vi "Initialize.vi"(8 "error in (no error)":errorcluster, 11 "FLOM Settings in":T1={"VISA resource name"="", "Simulated?"=FALSE, "Pump Number"=1.0} {"Pump Number" min=1.0 max=20.0 step=1.0}) -> (0 "error out":errorcluster, 1 "Initialized":bool, 2 "No Pump Connected":bool, 3 "FLOM Settings out":T1={"VISA resource name"="", "Simulated?"=FALSE, "Pump Number"=1.0} {"Pump Number" min=1.0 max=20.0 step=1.0})   [LabVIEW 2018, in "FLOM Pump.lvlib"]
uses:
  FLOM Pump.lvlib
  Settings Cluster.ctl
  <vilib>/Instr/_visa.llb/VISA Configure Serial Port (Instr).vi
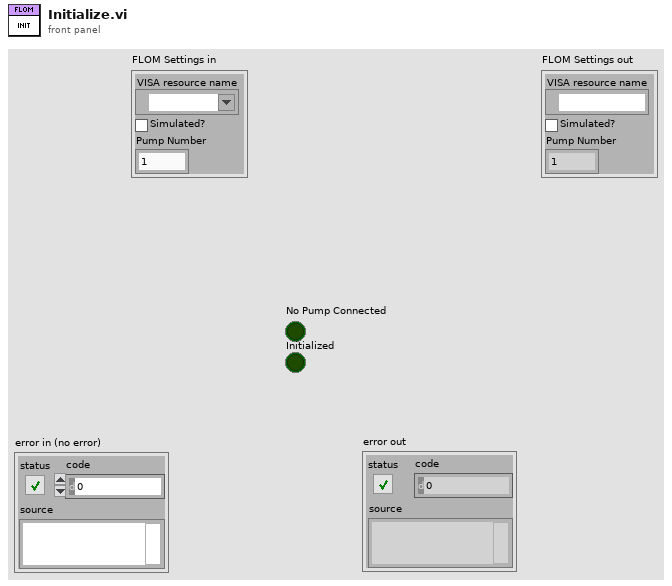
[diagram p1: front panel]
types:
  T1 = typedef "FLOM Pump.lvlib/Settings Cluster.ctl" = cluster{"VISA resource name":refnum<visa-resource-name>, "Simulated?":bool, "Pump Number":dbl}
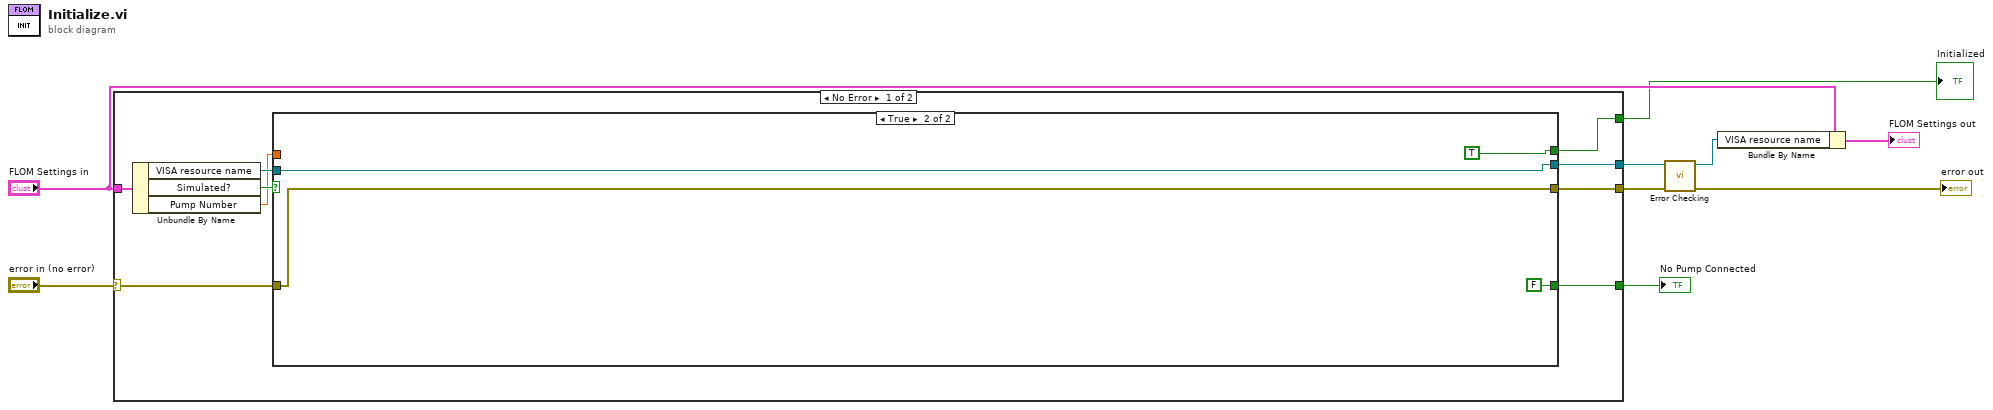
[diagram p0: block diagram]
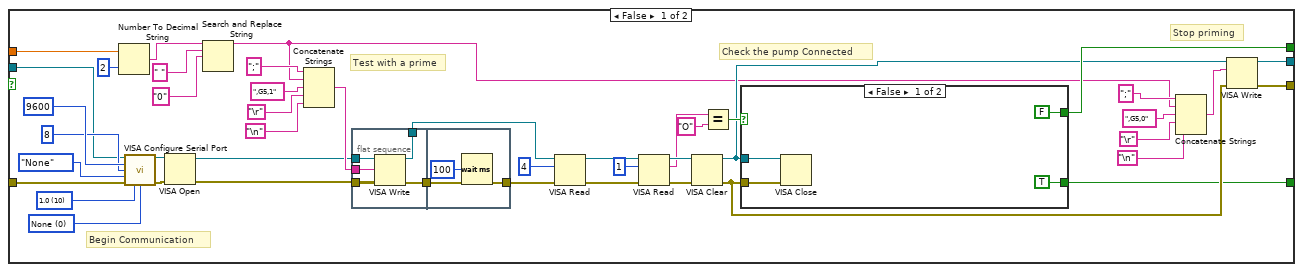
[diagram p2: hidden frame]
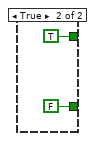
[diagram p3: hidden frame]
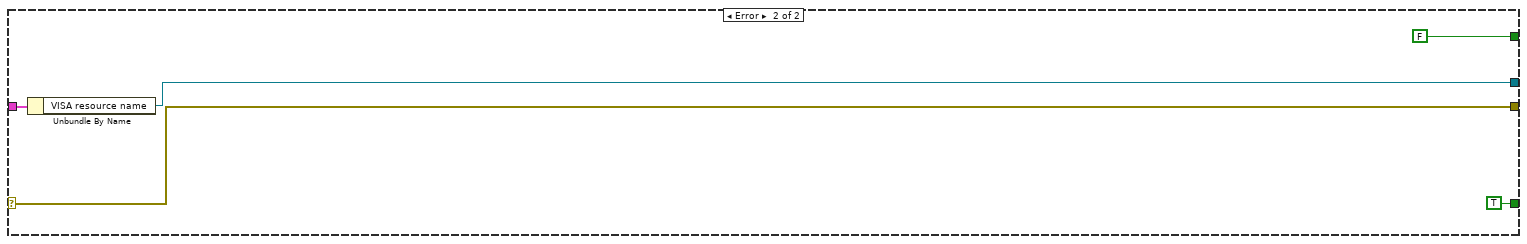
[diagram p4: hidden frame]
diagram:
  n1 = case shown="No Error" "error in (no error)" {
    selector: "error in (no error)" -> [w18 w85]
    tunnel: "FLOM Settings in" -> [w13 w84]
    tunnel: [w14 w85] -> w7
    tunnel: [w12 w83] -> w2
    tunnel: [w11 FALSE] -> w4
    tunnel: [w10 TRUE] -> w1
    frame No Error {
      n2 = Unbundle By Name(w13) -> ("VISA resource name"=w16:refnum<visa-resource-name>, "Simulated?"=w17:bool, "Pump Number"=w15:dbl)
      n3 = case shown="True" w17 {
        tunnel: w18 -> [w57 w80]
        tunnel: w16 -> [w55 w79]
        tunnel: w15 -> [w52 _]
        tunnel: [w22 w80] -> w14
        tunnel: [w20 w79] -> w12
        tunnel: [w47 TRUE] -> w11
        tunnel: [w19 FALSE] -> w10
        frame False {
          w59 = u16 0 items=["None", "XON/XOFF", "RTS/CTS", "XON/XOFF & RTS/CTS", "DTR/DSR", "XON/XOFF & DTR/DSR"] ("flow control (0:none)")
          w60 = u16 10 items=["1.0"=10, "1.5"=15, "2.0"=20] ("stop bits (10: 1 bit)")
          # "Stop priming"
          # "Test with a prime"
          # "Check the pump Connected"
          # "Begin Communication"
          n4 = Number To Decimal String(number=w52, width (-)=i16 2) -> (decimal integer string=w35:string)
          n5 = call-poly "VISA Configure Serial Port"("VISA resource name"=w55, "baud rate (9600)"=u32 9600, "data bits (8)"=u16 8, "parity (0:none)"=enum16{"None", "Odd", "Even", "Mark", "Space"}."None", "error in (no error)"=w57, "stop bits (10: 1 bit)"=w60, "flow control (0:none)"=w59) -> ("VISA resource name out"=w56:refnum<visa-resource-name>, "error out"=w58:errorcluster)  [unwired: 7 in]
          n6 = VISA Open(error in (no error)=w58, VISA resource name=w56) -> (VISA resource name=w31:refnum<visa-resource-name>, error out=w46:errorcluster)  [unwired: 3 in]
          n7 = Search and Replace String(input string=w35, search string=" ", replace string="0" ("replace string (\"\")")) -> (result string=w21:string)  [unwired: 5 in, 3 out]
          n8 = Concatenate Strings(";" ("string"), w21, ",G5,1" ("string"), "\r", "\n") -> (w53:string)
          n9 = flat-sequence {
            tunnel: w53 -> [w68]
            tunnel: w46 -> [w66]
            tunnel: [w67] -> w32
            tunnel: w31 -> [w65]
            tunnel: [w64] -> w30
            tunnel: [w70] -> w50
            tunnel: w32 -> [w70]
            frame #0 {
              n10 = VISA Write(VISA resource name=w65, write buffer=w68, error in (no error)=w66) -> (VISA resource name out=w64:refnum<visa-resource-name>, error out=w67:errorcluster)  [unwired: 1 out]
            }
            frame #1 {
              n11 = Wait (ms)(milliseconds to wait=u32 100) -> ()  [unwired: 1 out]
            }
          }
          n12 = VISA Read(VISA resource name=w30, byte count=u32 4, error in (no error)=w50) -> (VISA resource name out=w42:refnum<visa-resource-name>, error out=w41:errorcluster)  [unwired: 2 out]
          n13 = VISA Read(VISA resource name=w42, byte count=u32 1, error in (no error)=w41) -> (VISA resource name out=w40:refnum<visa-resource-name>, read buffer=w38:string, error out=w39:errorcluster)  [unwired: 1 out]
          n14 = VISA Clear(VISA resource name=w40, error in (no error)=w39) -> (VISA resource name out=w24:refnum<visa-resource-name>, error out=w23:errorcluster)
          n15 = Equal?(x=w38, y="O") -> (x = y?=w49:bool)
          n16 = case shown="False" w49 {
            tunnel: w24 -> [w74 _]
            tunnel: w23 -> [w73 _]
            tunnel: [TRUE FALSE] -> w19
            tunnel: [FALSE TRUE] -> w47
            frame False {
              n17 = VISA Close(VISA resource name=w74, error in (no error)=w73) -> ()  [unwired: 1 out]
            }
            frame True {
            }
          }
          n18 = Concatenate Strings(";" ("string"), w21, ",G5,0" ("string"), "\r", "\n") -> (w29:string)
          n19 = VISA Write(VISA resource name=w24, write buffer=w29, error in (no error)=w23) -> (VISA resource name out=w20:refnum<visa-resource-name>, error out=w22:errorcluster)  [unwired: 1 out]
        }
        frame True {
        }
      }
    }
    frame Error {
      n20 = Unbundle By Name(w84) -> ("VISA resource name"=w83:refnum<visa-resource-name>)
    }
  }
  "Initialized" <- w4
  "No Pump Connected" <- w1
  n21 = call "Error Checking.vi"("error in (no error)"=w7, "VISA resource name"=w2) -> ("error out"=→"error out":errorcluster, "VISA resource name"=w8:refnum<visa-resource-name>)  [unwired: 7 in, 1 out]
  n22 = Bundle By Name(cluster="FLOM Settings in", "VISA resource name"=w8) -> (→"FLOM Settings out":T1)
